vi "AlliGator Launcher.vi"() -> ()   [LabVIEW 2021, in "AlliGator GUI.lvlib"]
doc: "Runs transparently.\nLaunches AlliGator in transparent mode until initialization is complete."
uses:
  AlliGator GUI.lvlib
  Globals, Variables, Constants/AlliGator Variables List.ctl
  Notebook/Notebook Parameters List.ctl
  Globals, Variables, Constants/AlliGator Globals.vi
  AlliGator Check Version.vi
  AlliGator.vi
  Variant/Variant to Data/Variant to Boolean.vi
  Globals, Variables, Constants/AlliGator Globals, Variables & Constants.lvlib
  Variant/Variant to Data/Variant to Data.lvlib
  Notebook/Notebook.lvlib
  Utilities/Utilities.lvlib
  Action Engine/AlliGator Action Engine.lvlib
  Error/Error.lvlib
  <userlib>/_OpenG.lib/array/array.llb/openg_array.lvlib
  <userlib>/_OpenG.lib/array/array.llb/Filter 1D Array (String)__ogtk.vi
panel:
  out "About Message":string="© 2015-2023 The Regents of University of California\nAuthor: X. Michalet, Department of Chemistry & Biochemistry, UCLA\n\nThis software product was developed using LabVIEW™ and the National Instruments Vision Development Toolkit for LabVIEW. LabVIEW is a trademark of National Instruments.\n\nFunding was provided in part by grants from the US National Institute of Health, US Department of Energy, UC Cancer Research Coordination Committee and the UCLA Jonsson Comprehensive Cancer Center. AlliGator is not endorsed by, or sponsored by any of the above organizations.\n\nThis software is provided without guaranty of any kind, whether expressed or implied."
  out "Message":string
  out "Version":string
  out "Alligator":string="  AlliGator"
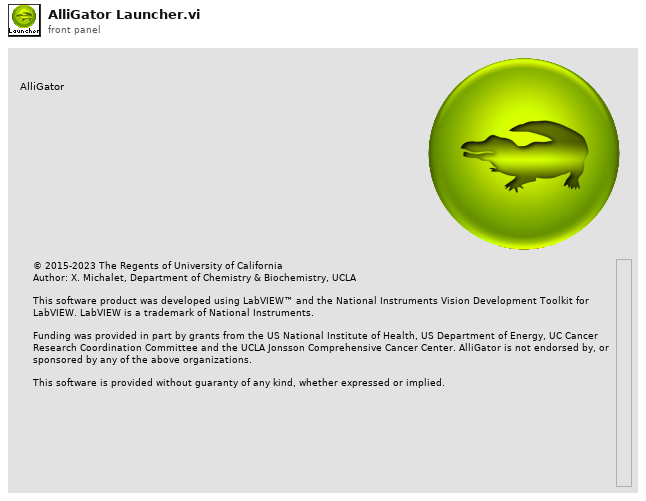
[diagram p1: front panel]
types:
  T1 = typedef "Notebook.lvlib/Notebook Parameters List.ctl" = enum16{"First Opening?", "Saved Notebook?", "Saved Notebook Path", "Beep on Error?"}
  T2 = enum32{"Invalid", "Standard", "Closed", "Hidden", "Minimized", "Maximized"}
  T3 = enum32{"Bad", "Idle", "Run top level", "Running"}
  T4 = typedef "AlliGator Globals, Variables & Constants.lvlib/AlliGator Variables List.ctl" = enum16{"---- GUI ----", "GUI:Initialization Status", "GUI:State Indicators Refnum", "GUI:Original AlliGator Menu Items", "GUI:Current Action Loop State", "GUI:Script in progress", "GUI:Playback", "GUI:Loop Playback", "GUI:Search ROI Used", "GUI:Search ROI", "Decay Graph Max Legend Size", "Intensity Graph Max Legend Size", "Decay Statistics Graph Max Legend Size", "Phasor Graph Max Legend Size", "Phasor Ratio Graph Max Legend Size", "Lifetime Graph Max Legend Size", "---- Files ----", "Files:Export Dataset Frames as Individual Files", "Files:Show Batch Export Help Balloons", "Files:Frames in Dataset", "Files:ptu File Frame Start Indices", "Files:Current Frame in Dataset", "Files:Current Frame Timestamp", "Files:Dataset Loaded", "Files:Dataset Metadata", "Files:Dataset Channel", "Files:Dataset Data Description", "Files:Background Dataset Metadata", "Files:Background Dataset Channel", "Files:Background Dataset Data Description", "Files:Background File Subtraction", "Files:Background File Path", "Files:Background File Pile-up Correction", "Files:Background File Pixel Well Capacity", "Files:Background File Scaling Factor", "Files:Current Dataset Load Settings", "Files:Dataset Path", "Files:ICCD-specific Information", "Files:Macrotime Gate Separation", "------ Python Plugins ------", "Python Plugins:Information", "Python Plugins:Python Session", "Python Plugins:Valid Python Session?", "---- Source Image ----", "Source Image:ROIs", "Source Image:Current ROI", "Source Image:ROI Event Refnum", "X_Source Image:Display Range", "X_Source Image:Palette Information", "X_Source Image:Type of Displayed Image", "X_Time Gate Slider", "Source Image:Palette List", "Source Image:Scale", "Source Image:ROI Overlay Color", "Source Image:Overlay to Erase", "Source Image:Is Displayed Image Accumulated", "Source Image:White Light Image Modified", "Source Image:Mask Image Modified", "---- Image Profile Window ----", "Image Profile:Window Event Refnum", "Image Profile:IntensityType", "Image Profile:Intensity Average Type", "Image Profile:Intensity-weighted SDV", "Image Profile:Box Profile Type", "Image Profile:Window Open", "Image Profile:Plotted Fit Parameter", "------ Phasor Graph -------", "Phasor Graph:Show Line", "---- Phasor Plot ---", "Phasor Plot:Parameters Changed", "Phasor Plot:FLI Dataset Modified since last Calculation", "Phasor Harmonics Data", "Selected Phasor Harmonics", "Phasor Harmonic Manager Event Refnum", "Phasor Plot:ROIs", "Phasor Plot:Current ROI", "Phasor Plot:ROI Event Refnum", "Phasor Plot:Image Reference Points", "Phasor Plot:Computed", "Phasor Plot:Palette Information", "Phasor Plot:Palette List", "Phasor Plot:Phasor Ratio Palette Information", "Phasor Plot:Phasor Ratio Palette List", "Phasor Plot:Image Scale", "Phasor Plot:Image Overlay to Erase", "Phasor Plot:Image Elements to Update", "Phasor Plot:Current Calculation Parameters", "Phasor Plot:Current Calibration Options", "Phasor Plot:Reset Cumulated Phasor Plot", "Phasor Plot:Reference 1", "Phasor Plot:Lifetime Reference 1", "Phasor Plot:Reference 1 Frequency", "Phasor Plot:Reference 2", "Phasor Plot:Lifetime Reference 2", "Phasor Plot:Reference 2 Frequency", "---- Decay Analysis ----", "Number of Selected Decays to Fit", "LS Fit Results", "LAR Fit Results", "BS Fit Results", "Last Decay Max - Min", "Best Fit Parameters", "Best Fit Parameter Names", "Actual Size X", "Actual Size Y", "Binning X", "Binning Y", "Actual # Gates", "Dataset Number", "Gates to...", "Gates Skipped", "Gates to keep", "Gate Step", "Gate Separation", "Reversed Gates", "Pile-up Correction", "Pixel Well Capacity", "Background Subtracted", "Background Subtraction Method", "Background Definition Range", "Background File (deprecated)", "Number of Dataset Accumulated", "Array of Accumulated Dataset Paths", "Do Averaged Datasets", "Destination File Path", "Process Plot Target", "Use 1/D as Phasor Frequency", "---- Decay Fit Parameter Map -----", "Decay Fit Parameter Map:Palette Information", "Decay Fit Parameter Map:Palette List", "Decay Fit Parameter Map:X Resolution", "Decay Fit Parameter Map:Y Resolution", "---- Parameter Map ----", "Parameter Map:Palette Information", "Parameter Map:Palette List", "------- Local Decay Window ---------", "Local Decay Graph Window:Event Refnum", "Local Decay Graph Window:Use normalized IRF for convolution", "----- Miscellaneous ----", "Misc:Skippable Dialog Windows Status"}
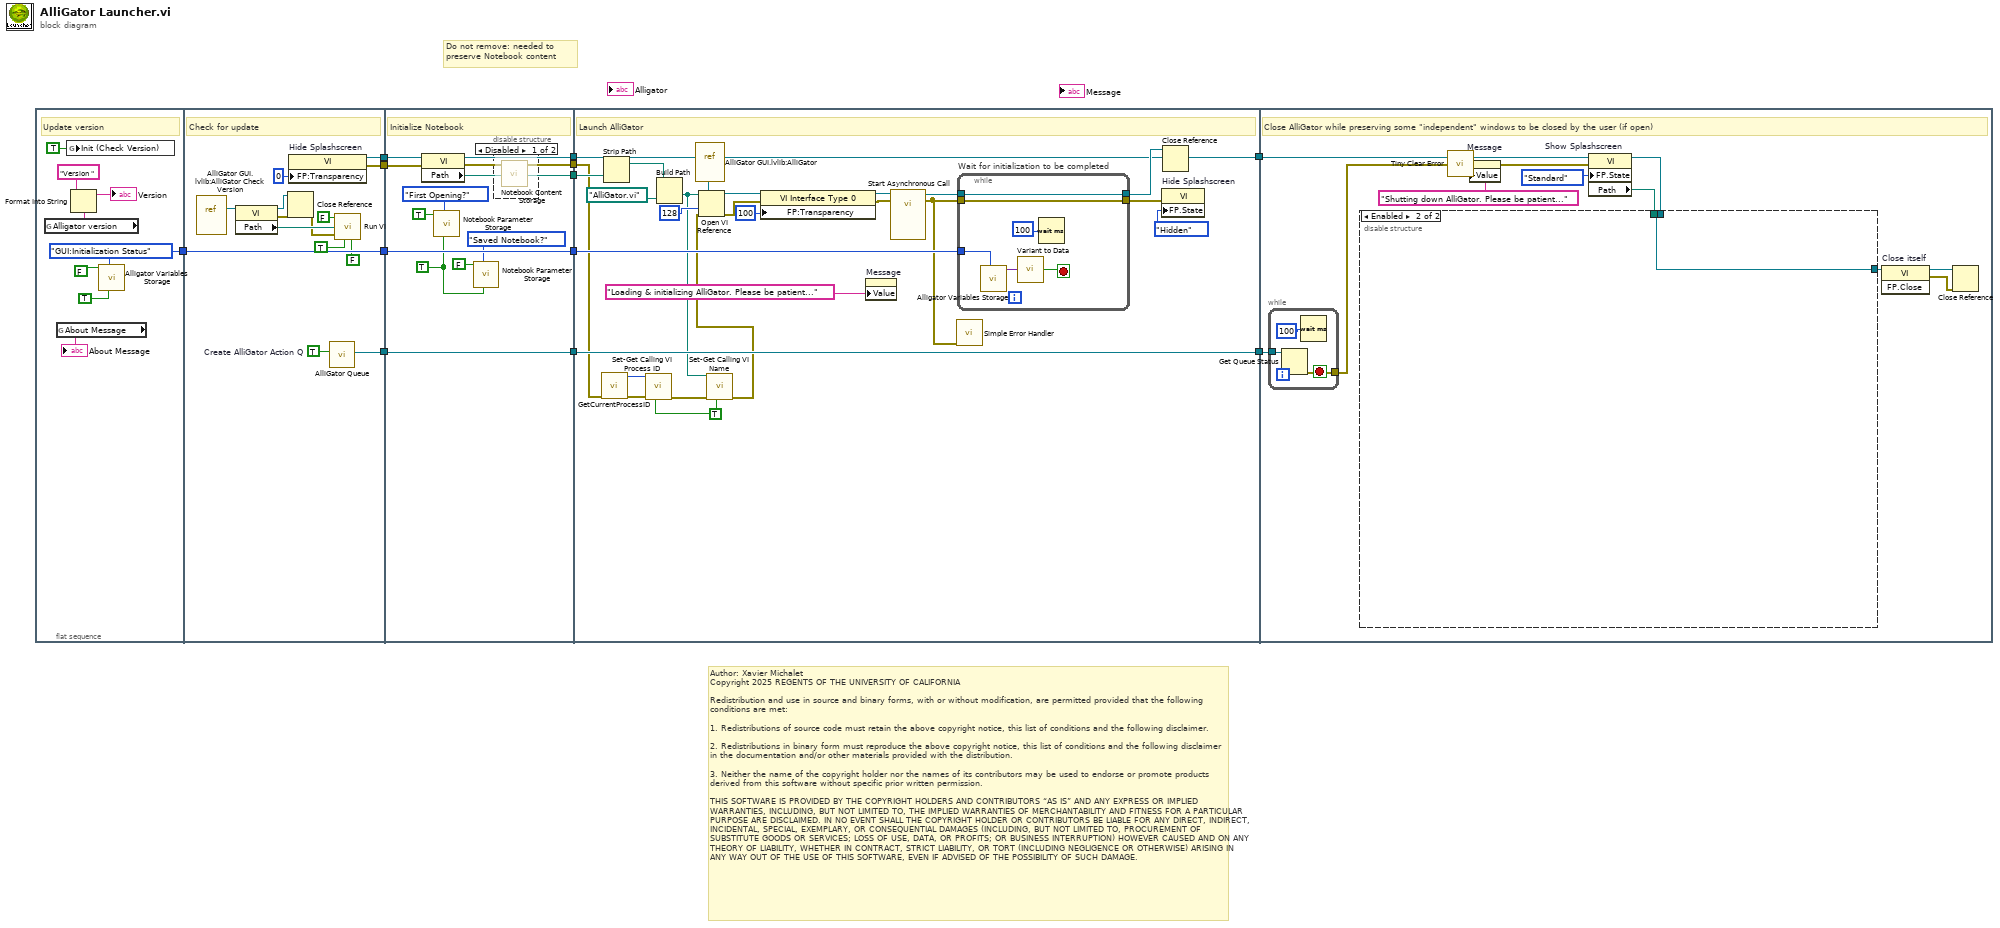
[diagram p0: block diagram]
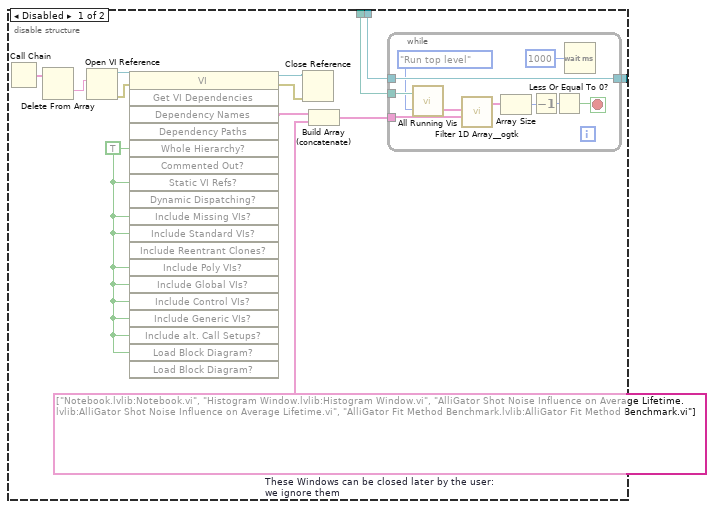
[diagram p3: hidden frame]
diagram:
  # "Author: Xavier Michalet\nCopyright 2025 REGENTS OF THE UNIVERSITY OF CALIFORNIA\n\nRedistribution and use in source and binary forms, with or without modification, are permitted provided that the following conditions are met:\n\n1. Redistributions of source code must retain the above copyright notice, this list of conditions and the following disclaimer.\n\n2. Redistributions in binary form must reproduce the above copyright notice, this list of conditions and the following disclaimer in the documentation and/or other materials provided with the distribution.\n\n3. Neither the name of the copyright holder nor the names of its contributors may be used to endorse or promote products derived from this software without specific prior written permission.\n\nTHIS SOFTWARE IS PROVIDED BY THE COPYRIGHT HOLDERS AND CONTRIBUTORS “AS IS” AND ANY EXPRESS OR IMPLIED WARRANTIES, INCLUDING, BUT NOT LIMITED TO, THE IMPLIED WARRANTIES OF MERCHANTABILITY AND FITNESS FOR A PARTICULAR PURPOSE ARE DISCLAIMED. IN NO EVENT SHALL THE COPYRIGHT HOLDER OR CONTRIBUTORS BE LIABLE FOR ANY DIRECT, INDIRECT, INCIDENTAL, SPECIAL, EXEMPLARY, OR CONSEQUENTIAL DAMAGES (INCLUDING, BUT NOT LIMITED TO, PROCUREMENT OF SUBSTITUTE GOODS OR SERVICES; LOSS OF USE, DATA, OR PROFITS; OR BUSINESS INTERRUPTION) HOWEVER CAUSED AND ON ANY THEORY OF LIABILITY, WHETHER IN CONTRACT, STRICT LIABILITY, OR TORT (INCLUDING NEGLIGENCE OR OTHERWISE) ARISING IN ANY WAY OUT OF THE USE OF THIS SOFTWARE, EVEN IF ADVISED OF THE POSSIBILITY OF SUCH DAMAGE."
  # "Do not remove: needed to preserve Notebook content"
  n1 = flat-sequence {
    tunnel: [w17] -> w12
    tunnel: [w34] -> w11
    tunnel: w12 -> [w34]
    tunnel: [w32] -> w7
    tunnel: [w31] -> w6
    tunnel: [w30] -> w5
    tunnel: w11 -> [w46]
    tunnel: [w46] -> w10
    tunnel: [w45] -> w8
    tunnel: w7 -> [w45]
    tunnel: w6 -> [w44]
    tunnel: w5 -> [w43]
    tunnel: [w42] -> w4
    tunnel: [w41] -> w3
    tunnel: [w35] -> w1
    tunnel: w10 -> [w67]
    tunnel: [w57] -> w9
    tunnel: w8 -> [w57]
    tunnel: w4 -> [w49]
    tunnel: w3 -> [w56]
    tunnel: [w54] -> w2
    tunnel: w1 -> [w54]
    tunnel: w9 -> [w85]
    tunnel: w2 -> [w79]
    frame #0 {
      w17 = AlliGator_Variables_List."GUI:Initialization Status" ("Alligator Variable")
      # "Update version"
      n2 = global read "AlliGator Globals.vi" "Alligator version"() -> (w14:string)
      n3 = global read "AlliGator Globals.vi" "About Message"() -> (→"About Message":string)
      n4 = global write "AlliGator Globals.vi" "Init (Check Version)"(TRUE ("Init (Check Version)")) -> ()
      n5 = Format Into String(initial string="Version ", w14) -> (resulting string=→"Version":string)  [unwired: 2 in, 1 out]
      n6 = call "Alligator Variables Storage.vi"("Get(F)/Set"=TRUE, "AlliGator Variable"=w17, "Data in"=FALSE ("Get(F)/Set")) -> ()  [unwired: 6 in, 3 out]
    }
    frame #1 {
      w21 = TRUE  # Create AlliGator Action Q
      # "Check for update"
      n7 = vi-ref "AlliGator GUI.lvlib:AlliGator Check Version.vi"() -> (w29:refnum<vi>)
      n8 = property class="VI"(reference=w29) -> (reference out=w24:refnum<vi>, error out=w23:errorcluster, "Path"=w28:path)  [unwired: 1 in]
      n9 = Close Reference(reference=w24, error in (no error)=w23) -> (error out=w22:errorcluster)
      n10 = property on="Hide Splashscreen" class="VI"("FP:Transparency"=u8 0 ("Front Panel Window:Transparency")) -> (reference out=w31:refnum<vi>, error out=w30:errorcluster)  [unwired: 2 in]
      n11 = call "AlliGator Queue.vi"("create if not found? (F)"=w21) -> ("AlliGator Q"=w32:refnum<queue>)  [unwired: 7 in, 1 out]
      n12 = call "Run Vi.vi"("Bring To Front (T)"=FALSE, "VI Path"=w28, "error in (no error)"=w22, "Start Hidden? (F)"=TRUE, "Activate? (T)"=FALSE) -> ()  [unwired: 3 in, 2 out]
    }
    frame #2 {
      w36 = TRUE ("Get(F)/Set")
      # "Initialize Notebook"
      n13 = property class="VI"(reference=w44, error in=w43) -> (reference out=w35:refnum<vi>, error out=w42:errorcluster, "Path"=w41:path)
      n14 = call "Notebook Parameter Storage.vi"("Get(F)/Set"=w36, "Notebook Parameter List"=Notebook_Parameters_List."First Opening?", "Data in"=TRUE ("Start Hidden? (F)")) -> ()  [unwired: 7 in, 2 out]
      n15 = call "Notebook Parameter Storage.vi"("Get(F)/Set"=w36, "Notebook Parameter List"=Notebook_Parameters_List."Saved Notebook?", "Data in"=FALSE ("Saved Notebook?")) -> ()  [unwired: 7 in, 2 out]
      n16 = disable-structure shown="Disabled" {
        frame Disabled {
          n17 = call "Notebook Content Storage.vi"() -> ()  [unwired: 10 in, 2 out]
        }
        frame Enabled {
        }
      }
    }
    frame #3 {
      w50 = TRUE ("Set/Get (F)")
      # "Launch AlliGator"
      n18 = call "GetCurrentProcessID.vi"("Error In"=w49) -> ("Error Out"=w51:errorcluster, "ProcessID"=w52:i32)  [unwired: 9 in]
      n19 = Strip Path(path=w56) -> (stripped path=w55:path)  [unwired: 1 out]
      n20 = call "Set-Get Calling VI Process ID.vi"("Set/Get (F)"=w50, "Error In"=w51, "ProcessID"=w52) -> ("Error Out"=w53:errorcluster)  [unwired: 7 in, 1 out]
      n21 = Build Path(base path=w55, name or relative path=path "AlliGator.vi" ("vi path")) -> (appended path=w48:path)
      n22 = vi-ref "AlliGator GUI.lvlib:AlliGator.vi"() -> (w69:refnum<vi>)
      n23 = call "Set-Get Calling VI Name.vi"("Set/Get (F)"=w50, "Error In"=w53, "Calling VI Path"=w48) -> ("Error Out"=w47:errorcluster)  [unwired: 7 in, 1 out]
      n24 = Open VI Reference(type specifier VI Refnum (for type only)=w69, vi path=w48, options=128, error in (no error)=w47) -> (vi reference=w61:refnum<vi>, error out=w60:errorcluster)  [unwired: 2 in]
      n25 = property class="VI Interface Type 0"(reference=w61, error in=w60, "FP:Transparency"=u8 100 ("Front Panel Window:Transparency")) -> (reference out=w59:refnum<vi>, error out=w58:errorcluster)
      n26 = property on="Message" class="Str"("Value"="Loading & initializing AlliGator. Please be patient..." ("Message")) -> ()  [unwired: 2 in, 2 out]
      n27 = call-by-ref "Start Asynchronous Call"(reference=w59, error in=w58) -> (reference out=w71:refnum<vi>, error out=w65:errorcluster)  [unwired: 1 in]
      n28 = call <vilib>:"Simple Error Handler.vi"("error in (no error)"=w65) -> ()  [unwired: 4 in, 5 out]
      n29 = while "Wait for initialization to be completed" {
        tunnel: w71 -> [w77]
        tunnel: w65 -> [w76]
        tunnel: [w77] -> w66
        tunnel: [w76] -> w68
        tunnel: w67 -> [w75]
        stop <- w73 stop-if-true
        n30 = call "Alligator Variables Storage.vi"("AlliGator Variable"=w75) -> ("Data out"=w74:variant)  [unwired: 8 in, 2 out]
        n31 = call-poly "Variant to Data.vi"("Variant"=w74) -> ("Value"=w73:bool)  [unwired: 8 in]
        n32 = Wait (ms)(milliseconds to wait=u32 100) -> ()  [unwired: 1 out]
      }
      n33 = property on="Hide Splashscreen" class="VI"(error in=w68, "FP.State"=T2."Hidden" ("Front Panel Window:State")) -> ()  [unwired: 1 in, 2 out]
      n34 = Close Reference(reference=w66) -> ()  [unwired: 1 in, 1 out]
    }
    frame #4 {
      # "Close AlliGator while preserving some \"independent\" windows to be closed by the user (if open)"
      n35 = while {
        tunnel: w85 -> [w117]
        tunnel: [w116] -> w80
        stop <- w116 stop-if-true
        n36 = Get Queue Status(queue=w117) -> (error out=w116:errorcluster)  [unwired: 2 in, 7 out]
        n37 = Wait (ms)(milliseconds to wait=u32 100) -> ()  [unwired: 1 out]
      }
      n38 = call "Tiny Clear Error.vi"("Error In"=w80) -> ("no Error Out"=w84:errorcluster)  [unwired: 8 in]
      n39 = property on="Message" class="Str"(error in=w84, "Value"="Shutting down AlliGator. Please be patient..." ("Message")) -> (error out=w88:errorcluster)  [unwired: 1 in, 1 out]
      n40 = property on="Show Splashscreen" class="VI"(reference=w79, error in=w88, "FP.State"=T2."Standard" ("Front Panel Window:State")) -> (reference out=w83:refnum<vi>, "Path"=w81:path)  [unwired: 1 out]
      n41 = disable-structure shown="Enabled" {
        disable-tunnel: w83 -> [w103 w114]
        disable-tunnel: [w102 w114] -> w82
        disable-tunnel: w81 -> [w101 _]
        frame Disabled {
          w93 = string[] ["Notebook.lvlib:Notebook.vi", "Histogram Window.lvlib:Histogram Window.vi", "AlliGator Shot Noise Influence on Average Lifetime.lvlib:AlliGator Shot Noise Influence on Average Lifetime.vi", "AlliGator Fit Method Benchmark.lvlib:AlliGator Fit Method Benchmark.vi"]  # These Windows can be closed later by the user: we ignore them
          w96 = TRUE ("Whole Hierarchy?")
          n42 = Call Chain() -> (call chain=w92:string[])
          n43 = Delete From Array(array=w92) -> (deleted portion=w91:string)  [unwired: 2 in, 1 out]
          n44 = Open VI Reference(vi path=w91) -> (vi reference=w100:refnum<vi>, error out=w99:errorcluster)  [unwired: 5 in]
          n45 = invoke class="VI" method="Get VI Dependencies"(reference=w100, error in=w99, "Whole Hierarchy?"=w96, "Static VI Refs?"=w96, "Include Missing VIs?"=w96, "Include Standard VIs?"=w96, "Include Poly VIs?"=w96, "Include Global VIs?"=w96, "Include Control VIs?"=w96, "Include Generic VIs?"=w96, "Include alt. Call Setups?"=w96, "Load Block Diagram?"=w96) -> (reference out=w95:refnum<vi>, error out=w94:errorcluster, "Dependency Names"=w97:string[])  [unwired: 7 in, 16 out]
          n46 = Close Reference(reference=w95, error in (no error)=w94) -> ()  [unwired: 1 out]
          n47 = Build Array (concatenate)(w97, w93) -> (w98:string[])
          n48 = while {
            tunnel: w98 -> [w112]
            tunnel: w103 -> [w107]
            tunnel: [w107] -> w102
            tunnel: w101 -> [w106]
            stop <- w108 stop-if-true
            n49 = call "All Running Vis.vi"("Execution State (Run Top Level)"=T3."Run top level", "Calling Vi path"=w106) -> ("Runnning Vi Names"=w113:string[])  [unwired: 1 out]
            n50 = call-poly <userlib>:"Filter 1D Array__ogtk.vi"("items to filter"=w112, "array"=w113) -> ("filtered array"=w111:string[])  [unwired: 4 in, 1 out]
            n51 = Array Size(array=w111) -> (size(s)=w110:i32)
            n52 = Decrement(x=w110) -> (x-1=w109:i32)
            n53 = Less Or Equal To 0?(x=w109) -> (x <= 0?=w108:bool)
            n54 = Wait (ms)(milliseconds to wait=u32 1000) -> ()  [unwired: 1 out]
          }
        }
        frame Enabled {
        }
      }
      n55 = invoke on="Close itself" class="VI" method="FP.Close"(reference=w82) -> (reference out=w89:refnum<vi>, error out=w90:errorcluster)  [unwired: 2 in, 1 out]
      n56 = Close Reference(reference=w89, error in (no error)=w90) -> ()  [unwired: 1 out]
    }
  }
